vi "DAQSensor-16.vi"() -> ()   [LabVIEW 2016]
uses:
  <vilib>/Utility/error.llb/DialogType.ctl
  PLC-Lab/lib/gusb.dll
panel:
  in  "量程B 5":dbl=100.0
  in  "量程A 5":dbl
  in  "备注 5":string="CH5" caption="CH5"
  in  "选中 5":bool
  in  "量程B 6":dbl=100.0
  in  "量程A 6":dbl
  in  "备注 6":string="CH6" caption="CH6"
  in  "选中 6":bool
  in  "量程B 7":dbl=100.0
  in  "量程A 7":dbl
  in  "备注 7":string="CH7" caption="CH7"
  in  "选中 7":bool
  in  "量程B 8":dbl=100.0
  in  "量程A 8":dbl
  in  "备注 8":string="CH8" caption="CH8"
  in  "选中 8":bool
  in  "量程B 9":dbl=100.0
  in  "量程A 9":dbl
  in  "备注 9":string="CH9" caption="CH9"
  in  "选中 9":bool
  in  "量程B 10":dbl=100.0
  in  "量程A 10":dbl
  in  "备注 10":string="CH10" caption="CH10"
  in  "选中 10":bool
  in  "量程B 11":dbl=100.0
  in  "量程A 11":dbl
  in  "备注 11":string="CH11" caption="CH11"
  in  "选中 11":bool
  in  "量程B 12":dbl=100.0
  in  "量程A 12":dbl
  in  "备注 12":string="CH12" caption="CH12"
  in  "选中 12":bool
  in  "量程B 13":dbl=100.0
  in  "量程A 13":dbl
  in  "备注 13":string="CH13" caption="CH13"
  in  "选中 13":bool
  in  "量程B 14":dbl=100.0
  in  "量程A 14":dbl
  in  "备注 14":string="CH14" caption="CH14"
  in  "选中 14":bool
  in  "量程B 15":dbl=100.0
  in  "量程A 15":dbl
  in  "备注 15":string="CH15" caption="CH15"
  in  "选中 15":bool
  in  "量程B 16":dbl=100.0
  in  "量程A 16":dbl
  in  "备注 16":string="CH16" caption="CH16"
  in  "选中 16":bool
  in  "布尔":bool
  out "采集准备完成":bool
  out "PLC就绪":bool
  out "警告":bool
  out "故障":bool
  out "原位":bool
  out "R0":bool
  out "PLC状态":dbl
  out "实际备注数组":string[](array[string])
  out "通道数":u32
  in  "单位 2":string
  in  "单位 1":string
  in  "单位 3":string
  in  "单位 4":string
  in  "单位 5":string
  in  "单位 6":string
  in  "单位 7":string
  in  "单位 8":string
  in  "单位 9":string
  in  "单位 10":string
  in  "单位 11":string
  in  "单位 12":string
  in  "单位 13":string
  in  "单位 14":string
  in  "单位 15":string
  in  "单位 16":string
  out "系数":sgl[][](array[numeric])
  out "量程B数组":dbl[](array[numeric])
  out "量程A数组":dbl[](array[numeric])
  out "备注数组":string[](array[string])
  out "给采集卡的通道选择":i16
  in  "选项卡控件":enum32{"设置", "数据采集", "历史数据"}(tab)
  in  "最大采集时间(秒)":dbl=5.0 min=0.1 max=15.0
  in  "测试模式选择":enum32{"测试模式1", "测试模式2"}(radio)
  in  "数据存储":bool=TRUE
  in  "量程":u16=10 caption="传感器输出范围"
  in  "通道模式":enum32{"单选选项1", "单选选项2"}(radio)=enum."单选选项2"
  in  "电压电流选择":enum32{"单选选项1", "单选选项2"}(radio)
  in  "产品系列":u16(ring)=1 items=["USB-4000", "USB-2000/1000"]
  in  "传感器单位":string
  in  "数据存储路径":path=path "D:/采集存储/辅助锁力数据"
  in  "传感器输出范围B":dbl=5.0 caption="传感器输出范围"
  in  "传感器输出范围A":dbl caption="传感器输出范围"
  in  "采样率(Sps/s)":u32=500 step=5
  in  "设置生效":bool
  in  "全选":bool
  in  "量程B 2":dbl=100.0
  in  "量程A 2":dbl
  in  "备注 2":string="CH2" caption="CH2"
  in  "选中 2":bool=TRUE
  in  "量程B 1":dbl=100.0
  in  "量程A 1":dbl
  in  "备注 1":string="CH1" caption="CH1"
  in  "选中 1":bool=TRUE
  in  "量程B 3":dbl=100.0
  in  "量程A 3":dbl
  in  "备注 3":string="CH3" caption="CH3"
  in  "选中 3":bool=TRUE
  in  "量程B 4":dbl=100.0
  in  "量程A 4":dbl
  in  "备注 4":string="CH4" caption="CH4"
  in  "选中 4":bool
  in  "转角起点(0.1°)":i32=-350 min=-400 max=400
  in  "转角终点(0.1°)":i32=350 min=200 max=400
  in  "转角速度(转/min)":i32=50 min=10 max=70
  in  "气压设定(0.1MPa)":i32=5 min=2 max=10
  out "测量类型":i32 min=0 max=1
  out "波形图表":sgl[][](graph)
  in  "调用统计信息":bool
  in  "停止":bool
  in  "启动":bool
  in  "转为CSV":bool
  out "波形图表 2":sgl[][](graph)
  in  "历史数据路径":path
  in  "打开":bool
  # "单位"
  # "mA ~              mA"
  # "V ~                 V"
  # "Via Ruiwen"
  # "DAQSensor"
  # "请求原位"
  # "仅启动辅助锁"
  # "通道注释"
  # "传感器量程"
  # "仅USB-2000系列支持差分模式"
  # "~"
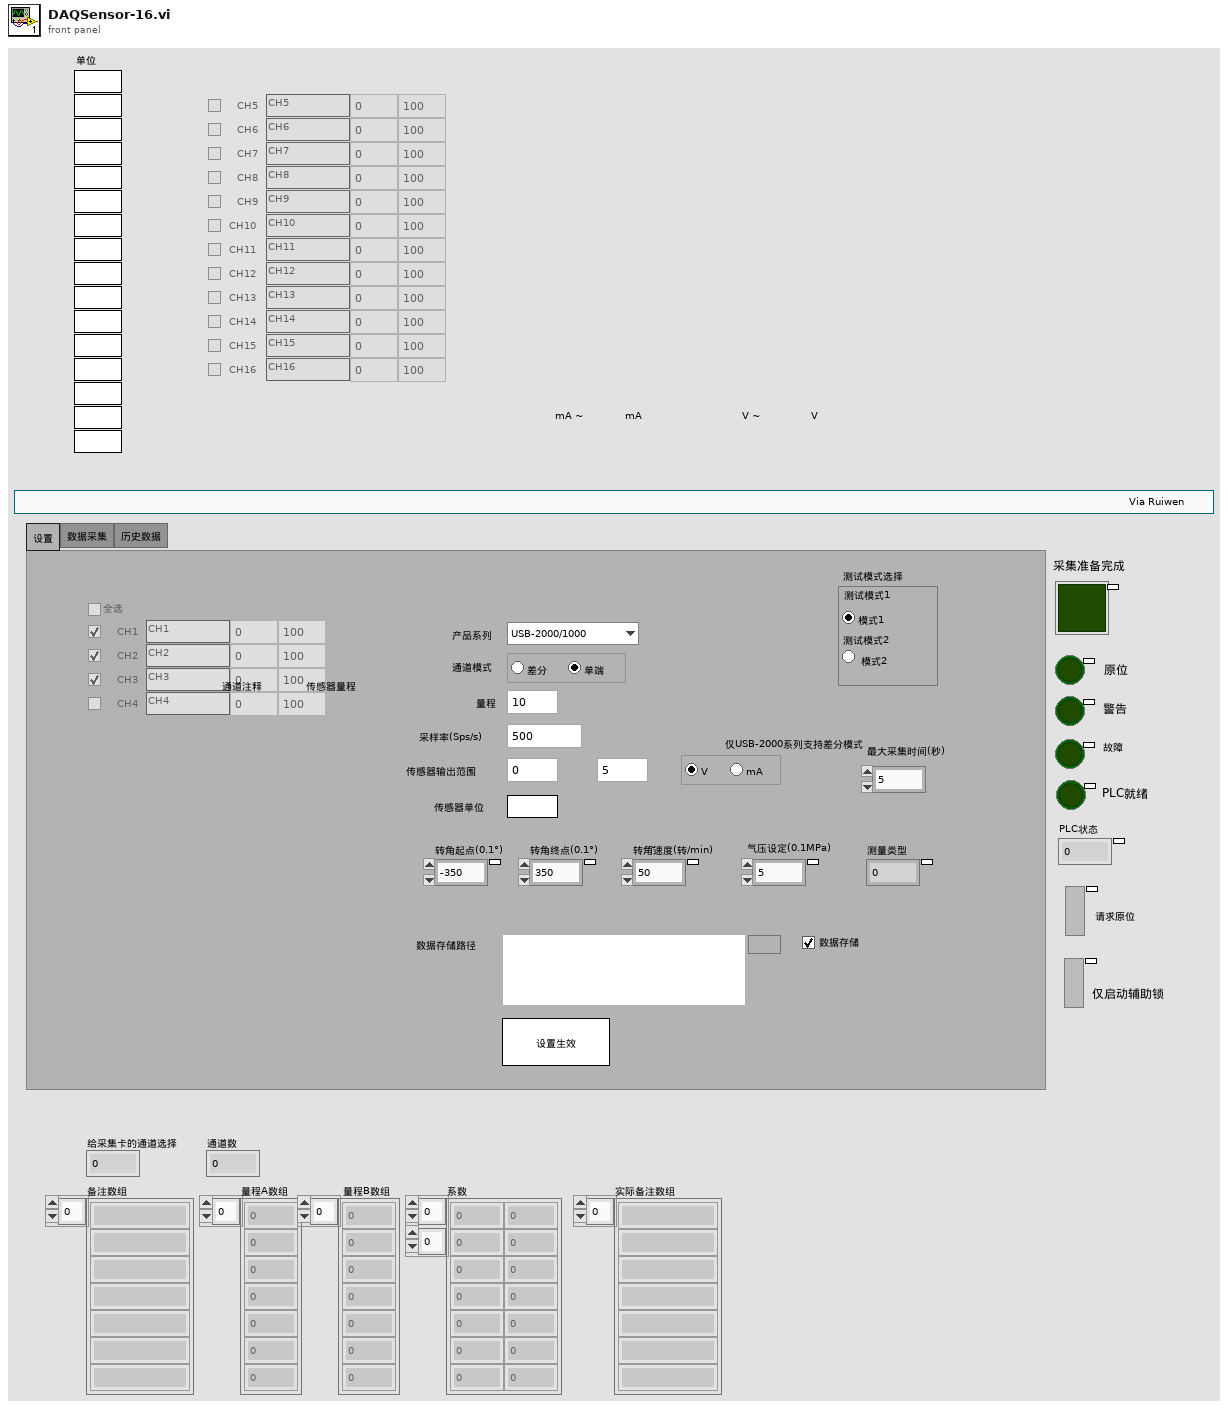
[diagram p1: front panel]
types:
  T1 = enum32{"Bad", "Idle", "Run top level", "Running"}
  T2 = enum8{"Enabled", "Disabled", "Disabled and Grayed Out"}
  T3 = cluster{"seconds since 1Jan1904":timestamp, "采样率":u32, "单位":string, "实际备注数组":string[]}
  T4 = typedef "DialogType.ctl" = u16
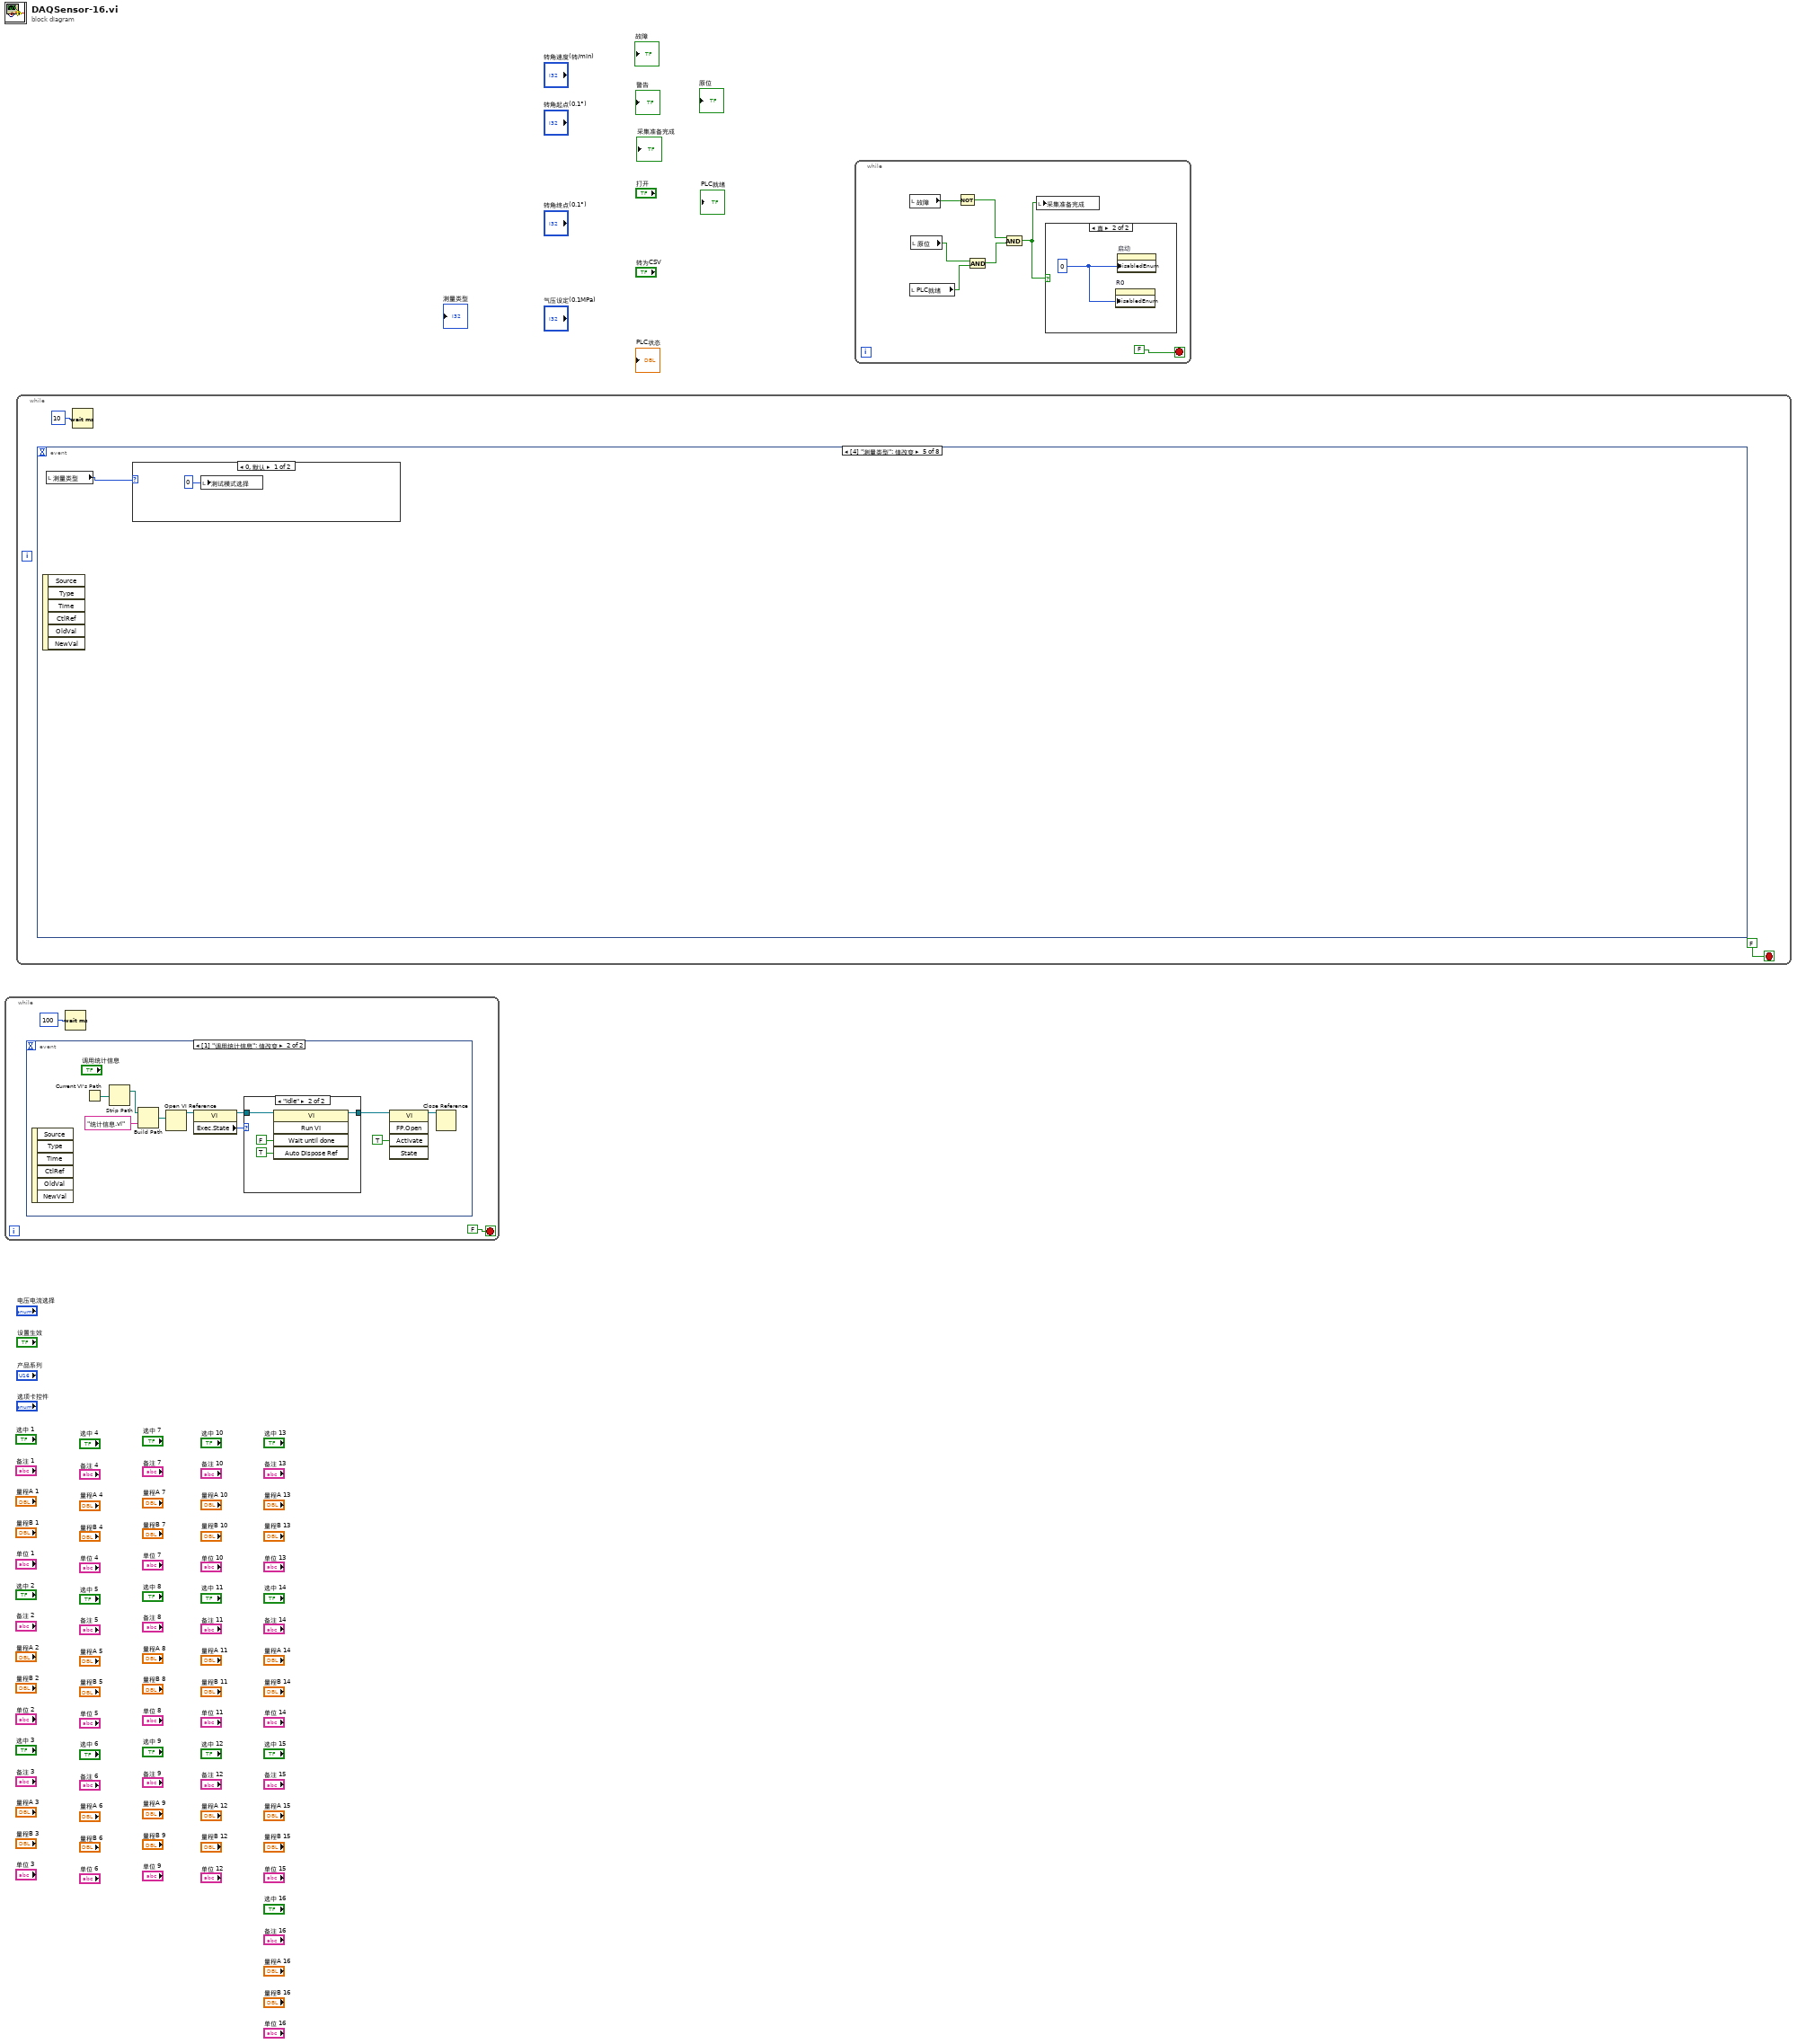
[diagram p0: block diagram]
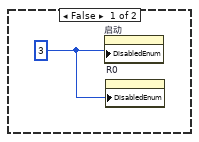
[diagram p2: hidden frame]
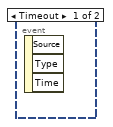
[diagram p3: hidden frame]
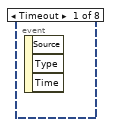
[diagram p5: hidden frame]
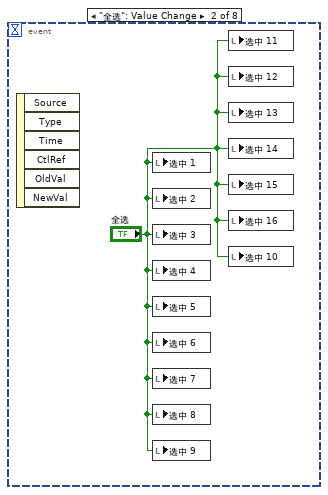
[diagram p6: hidden frame]
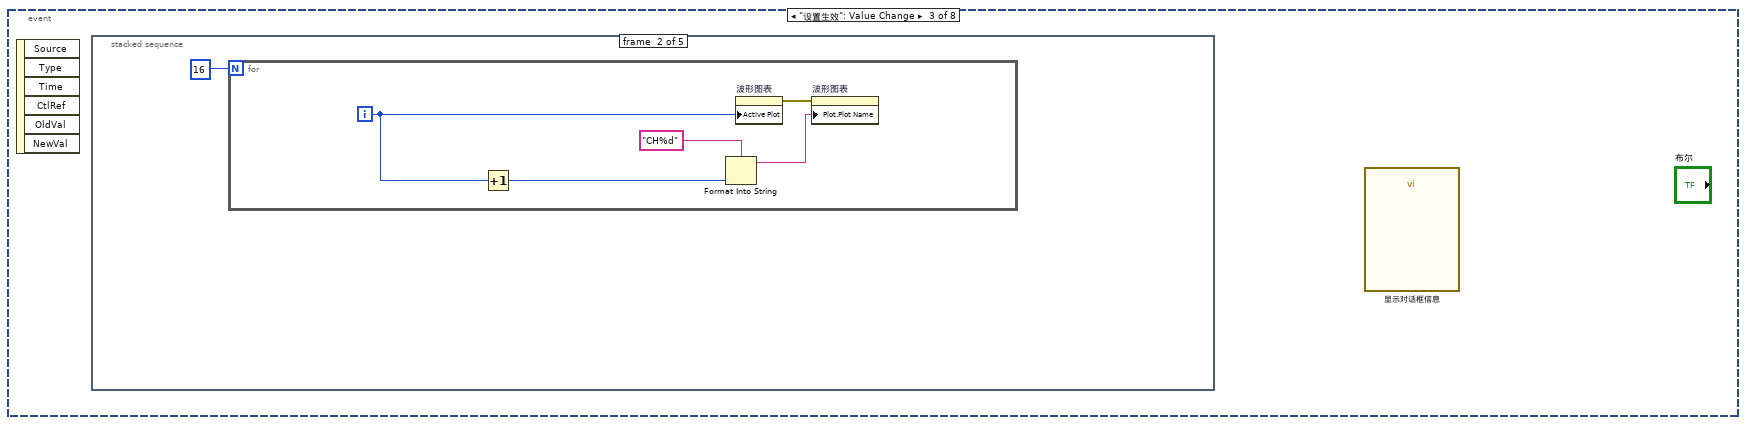
[diagram p7: hidden frame]
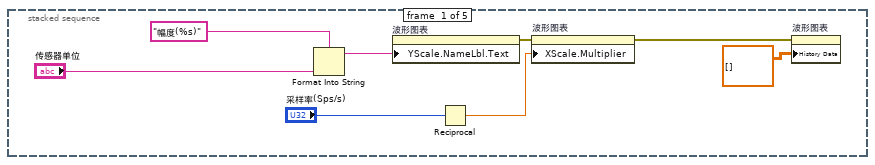
[diagram p8: hidden frame]
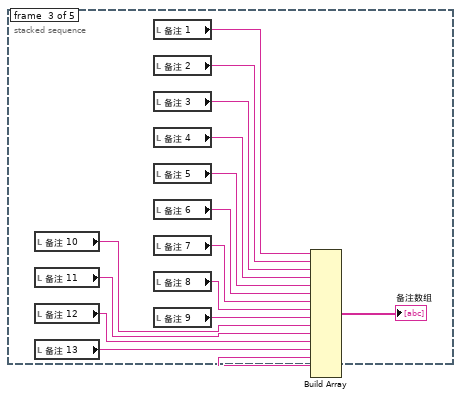
[diagram p9: hidden frame]
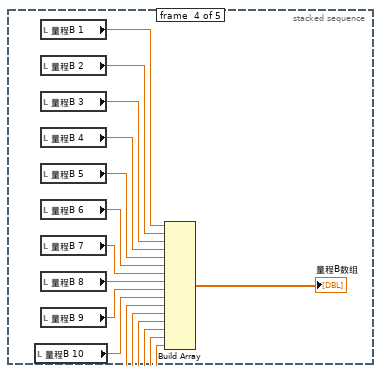
[diagram p10: hidden frame]
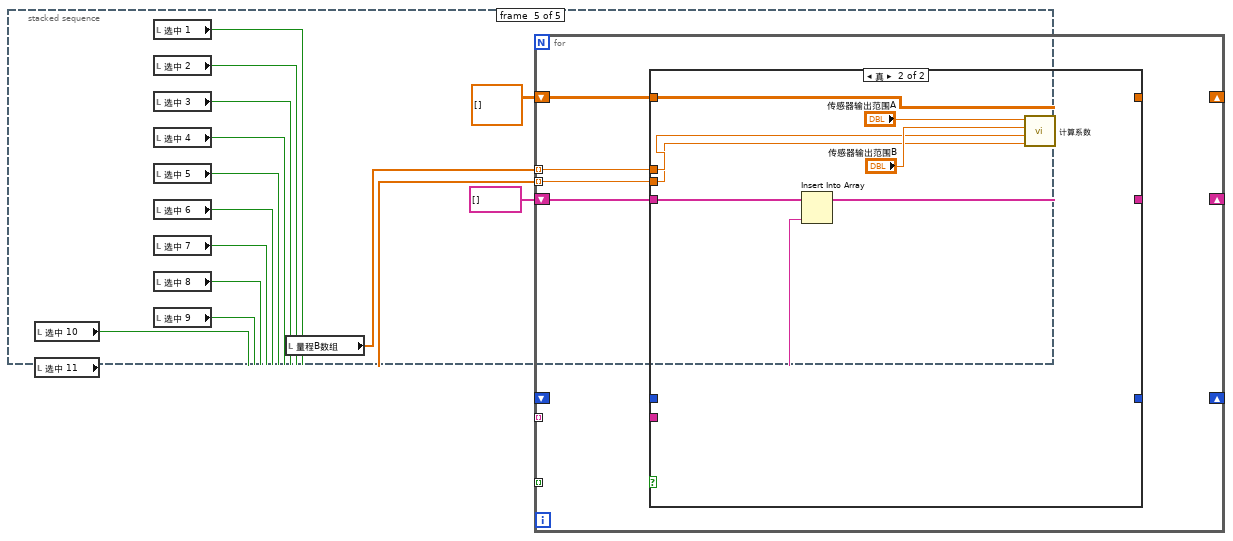
[diagram p11: hidden frame]
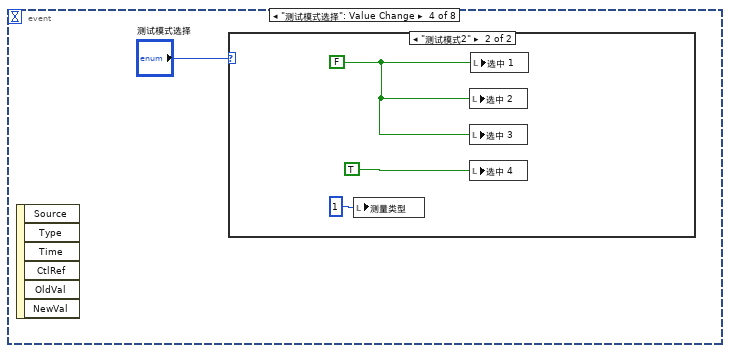
[diagram p13: hidden frame]
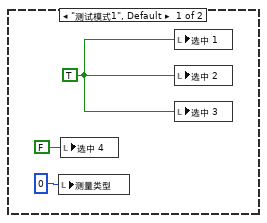
[diagram p14: hidden frame]
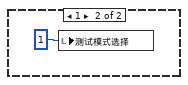
[diagram p15: hidden frame]
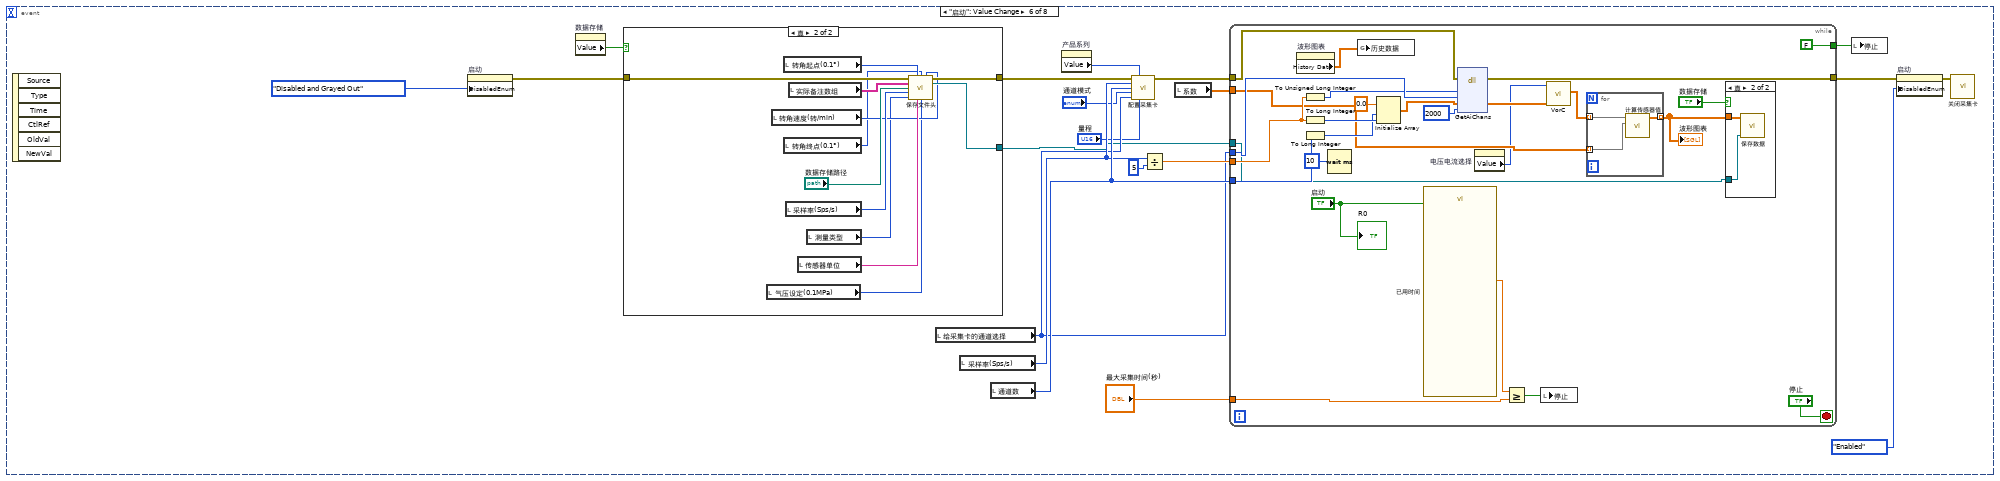
[diagram p16: hidden frame]
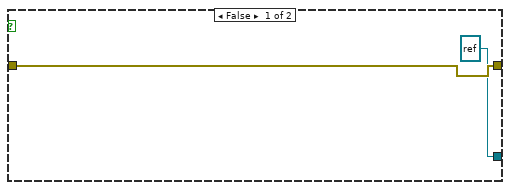
[diagram p17: hidden frame]
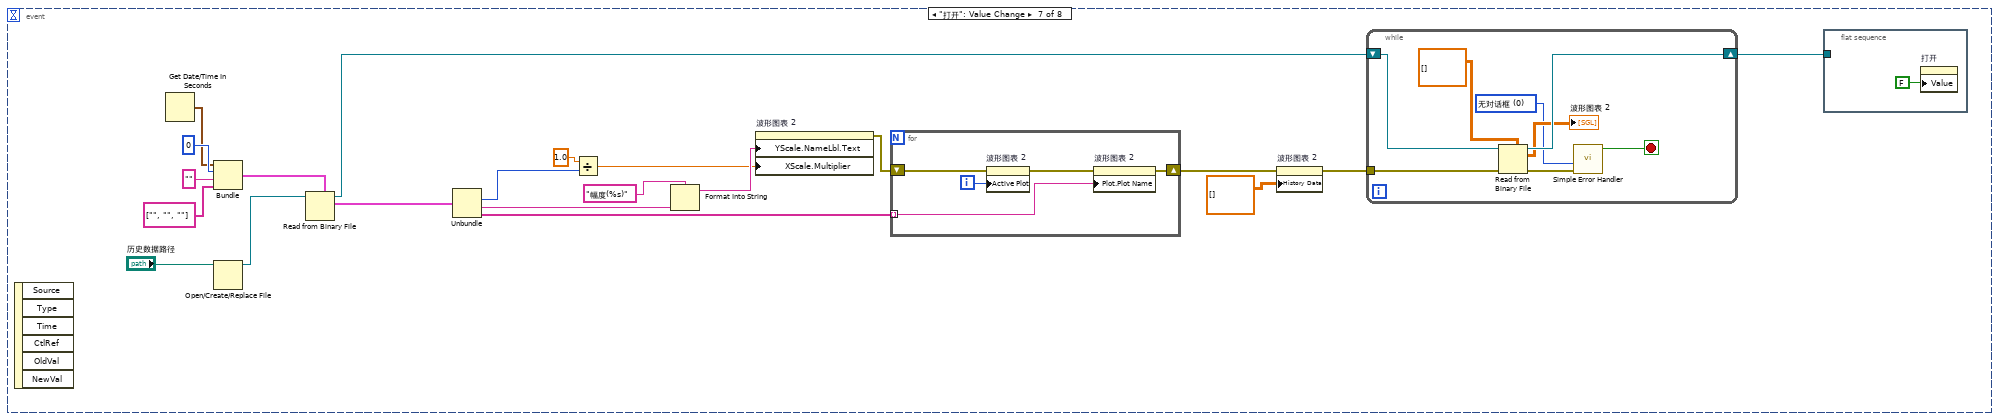
[diagram p19: hidden frame]
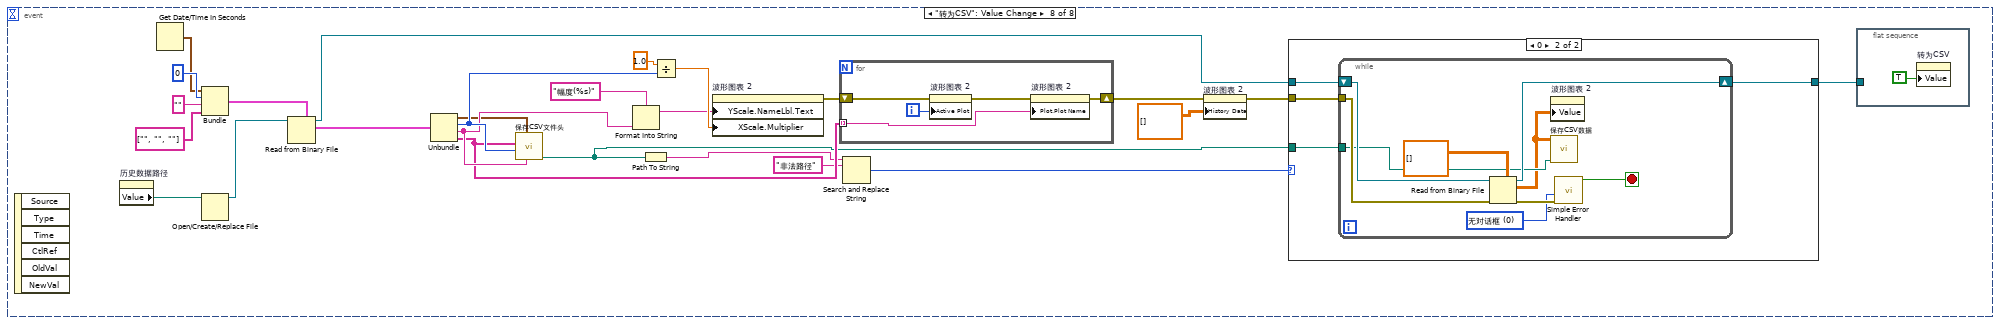
[diagram p20: hidden frame]
diagram:
  n1 = while {
    stop <- FALSE stop-if-true
    n2 = event shown="[1] \"调用统计信息\": 值改变" {
      selector: _ -> [_ _]
      dyn-events: _ -> [_ _]
      timeout: _ -> [_ _]
      event Timeout {
        n3 = event-data() -> ()  [unwired: 1 in, 3 out]
      }
      event "调用统计信息": Value Change {
        n4 = event-data() -> ()  [unwired: 1 in, 6 out]
        n5 = Current VI's Path() -> (path=w3:path)
        n6 = Strip Path(path=w3) -> (stripped path=w4:path)  [unwired: 1 out]
        n7 = Build Path(base path=w4, name or relative path="统计信息.vi" ("名称或相对路径")) -> (appended path=w5:path)
        n8 = Open VI Reference(vi path=w5) -> (vi reference=w6:refnum<vi>)  [unwired: 5 in, 1 out]
        n9 = property class="VI"(reference=w6) -> (reference out=w9:refnum<vi>, "Exec.State"=w7:T1)  [unwired: 1 in, 1 out]
        n10 = case shown="\"Idle\"" w7 {
          tunnel: [w13 w15] -> w8
          tunnel: w9 -> [w13 w14]
          frame "Bad", Default {
          }
          frame "Idle" {
            n11 = invoke class="VI" method="Run VI"(reference=w14, "Wait until done"=FALSE ("结束前等待"), "Auto Dispose Ref"=TRUE ("自动销毁引用")) -> (reference out=w15:refnum<vi>)  [unwired: 2 in, 4 out]
          }
        }
        n12 = invoke class="VI" method="FP.Open"(reference=w8, "Activate"=TRUE ("激活？")) -> (reference out=w11:refnum<vi>)  [unwired: 3 in, 4 out]
        n13 = Close Reference(reference=w11) -> ()  [unwired: 1 in, 1 out]
      }
    }
    n14 = Wait (ms)(milliseconds to wait=u32 100 ("等待时间（毫秒）")) -> ()  [unwired: 1 out]
  }
  n15 = while {
    stop <- FALSE stop-if-true
    n16 = event shown="[4] \"测量类型\": 值改变" {
      selector: _ -> [_ _ _ _ _ _ _ _]
      dyn-events: _ -> [_ _ _ _ _ _ _ _]
      timeout: _ -> [_ _ _ _ _ _ _ _]
      event Timeout {
        n17 = event-data() -> ()  [unwired: 1 in, 3 out]
      }
      event "全选": Value Change {
        n18 = event-data() -> ()  [unwired: 1 in, 6 out]
        n19 = local write "选中 1"("全选") -> ()
        n20 = local write "选中 2"("全选") -> ()
        n21 = local write "选中 3"("全选") -> ()
        n22 = local write "选中 4"("全选") -> ()
        n23 = local write "选中 5"("全选") -> ()
        n24 = local write "选中 6"("全选") -> ()
        n25 = local write "选中 7"("全选") -> ()
        n26 = local write "选中 8"("全选") -> ()
        n27 = local write "选中 9"("全选") -> ()
        n28 = local write "选中 11"("全选") -> ()
        n29 = local write "选中 12"("全选") -> ()
        n30 = local write "选中 13"("全选") -> ()
        n31 = local write "选中 14"("全选") -> ()
        n32 = local write "选中 15"("全选") -> ()
        n33 = local write "选中 16"("全选") -> ()
        n34 = local write "选中 10"("全选") -> ()
      }
      event "设置生效": Value Change {
        n35 = event-data() -> ()  [unwired: 1 in, 6 out]
        n36 = stacked-sequence {
          frame #0 {
            n37 = Format Into String(format string="幅度(%s)" ("格式字符串"), "传感器单位") -> (resulting string=w25:string)  [unwired: 2 in, 1 out]
            n38 = property on="波形图表" class="WFChart (严格)"("YScale.NameLbl.Text"=w25) -> (error out=w21:errorcluster)  [unwired: 2 in, 1 out]
            n39 = Reciprocal(x="采样率(Sps/s)") -> (1/x=w24:dbl)
            n40 = property on="波形图表" class="WFChart (严格)"(error in=w21, "XScale.Multiplier"=w24) -> (error out=w22:errorcluster)  [unwired: 1 in, 1 out]
            n41 = property on="波形图表" class="WFChart (严格)"(error in=w22, "History Data"=dbl[][] [] ("历史数据")) -> ()  [unwired: 1 in, 2 out]
          }
          frame #1 {
            n42 = for {
              N: 16 -> [_]
              i -> [w32]
              n43 = Increment(x=w32) -> (x+1=w33:i32)
              n44 = Format Into String(format string="CH%d" ("格式字符串"), w33) -> (resulting string=w30:string)  [unwired: 2 in, 1 out]
              n45 = property on="波形图表" class="WFChart (严格)"("Active Plot"=w32) -> (error out=w31:errorcluster)  [unwired: 2 in, 1 out]
              n46 = property on="波形图表" class="WFChart (严格)"(error in=w31, "Plot.Plot Name"=w30) -> ()  [unwired: 1 in, 2 out]
            }
          }
          frame #2 {
            n47 = local read "备注 10"() -> (w45:string)
            n48 = local read "备注 11"() -> (w46:string)
            n49 = local read "备注 12"() -> (w47:string)
            n50 = local read "备注 13"() -> (w48:string)
            n51 = local read "备注 14"() -> (w49:string)
            n52 = local read "备注 15"() -> (w50:string)
            n53 = local read "备注 16"() -> (w51:string)
            n54 = local read "备注 1"() -> (w36:string)
            n55 = local read "备注 2"() -> (w37:string)
            n56 = local read "备注 3"() -> (w38:string)
            n57 = local read "备注 4"() -> (w39:string)
            n58 = local read "备注 5"() -> (w40:string)
            n59 = local read "备注 6"() -> (w41:string)
            n60 = local read "备注 7"() -> (w42:string)
            n61 = local read "备注 8"() -> (w43:string)
            n62 = local read "备注 9"() -> (w44:string)
            n63 = Build Array(w36, w37, w38, w39, w40, w41, w42, w43, w44, w45, w46, w47, w48, w49, w50, w51) -> (→"备注数组":string[])
          }
          frame #3 {
            n64 = local read "量程B 10"() -> (w58:dbl)
            n65 = local read "量程B 11"() -> (w57:dbl)
            n66 = local read "量程B 12"() -> (w56:dbl)
            n67 = local read "量程B 13"() -> (w55:dbl)
            n68 = local read "量程B 14"() -> (w54:dbl)
            n69 = local read "量程B 15"() -> (w53:dbl)
            n70 = local read "量程B 16"() -> (w52:dbl)
            n71 = local read "量程A 10"() -> (w79:dbl)
            n72 = local read "量程A 11"() -> (w80:dbl)
            n73 = local read "量程A 12"() -> (w81:dbl)
            n74 = local read "量程A 13"() -> (w82:dbl)
            n75 = local read "量程A 14"() -> (w83:dbl)
            n76 = local read "量程A 15"() -> (w84:dbl)
            n77 = local read "量程A 16"() -> (w85:dbl)
            n78 = local read "量程B 1"() -> (w67:dbl)
            n79 = local read "量程B 2"() -> (w66:dbl)
            n80 = local read "量程B 3"() -> (w65:dbl)
            n81 = local read "量程B 4"() -> (w64:dbl)
            n82 = local read "量程B 5"() -> (w63:dbl)
            n83 = local read "量程B 6"() -> (w62:dbl)
            n84 = local read "量程B 7"() -> (w61:dbl)
            n85 = local read "量程B 8"() -> (w60:dbl)
            n86 = local read "量程B 9"() -> (w59:dbl)
            n87 = local read "量程A 1"() -> (w70:dbl)
            n88 = local read "量程A 2"() -> (w71:dbl)
            n89 = local read "量程A 3"() -> (w72:dbl)
            n90 = local read "量程A 4"() -> (w73:dbl)
            n91 = local read "量程A 5"() -> (w74:dbl)
            n92 = local read "量程A 6"() -> (w75:dbl)
            n93 = local read "量程A 7"() -> (w76:dbl)
            n94 = local read "量程A 8"() -> (w77:dbl)
            n95 = local read "量程A 9"() -> (w78:dbl)
            n96 = Build Array(w67, w66, w65, w64, w63, w62, w61, w60, w59, w58, w57, w56, w55, w54, w53, w52) -> (→"量程B数组":dbl[])
            n97 = Build Array(w70, w71, w72, w73, w74, w75, w76, w77, w78, w79, w80, w81, w82, w83, w84, w85) -> (→"量程A数组":dbl[])
          }
          frame #4 {
            n98 = local read "选中 10"() -> (w104:bool)
            n99 = local read "选中 11"() -> (w103:bool)
            n100 = local read "选中 12"() -> (w102:bool)
            n101 = local read "选中 13"() -> (w101:bool)
            n102 = local read "选中 14"() -> (w100:bool)
            n103 = local read "选中 15"() -> (w99:bool)
            n104 = local read "选中 16"() -> (w98:bool)
            n105 = local read "选中 1"() -> (w113:bool)
            n106 = local read "选中 2"() -> (w112:bool)
            n107 = local read "选中 3"() -> (w111:bool)
            n108 = local read "选中 4"() -> (w110:bool)
            n109 = local read "选中 5"() -> (w109:bool)
            n110 = local read "选中 6"() -> (w108:bool)
            n111 = local read "选中 7"() -> (w107:bool)
            n112 = local read "选中 8"() -> (w106:bool)
            n113 = local read "选中 9"() -> (w105:bool)
            n114 = local read "量程B数组"() -> (w91:dbl[])
            n115 = local read "量程A数组"() -> (w92:dbl[])
            n116 = local read "备注数组"() -> (w93:string[])
            n117 = Build Array(w113, w112, w111, w110, w109, w108, w107, w106, w105, w104, w103, w102, w101, w100, w99, w98) -> (w96:bool[])
            n118 = Boolean Array To Number(Boolean array=w96) -> (number=w97:u32)
            n119 = for {
              tunnel: w96 -> [w123] mode=indexing
              shift-right: [w121] -> w88
              shift-left: u32 0 -> [w122]
              tunnel: w93 -> [w120] mode=indexing
              tunnel: w92 -> [w119] mode=indexing
              tunnel: w91 -> [w118] mode=indexing
              shift-right: [w116] -> w89
              shift-left: dbl[][] [] -> [w117]
              shift-right: [w114] -> w86
              shift-left: string[] [] -> [w115]
              n120 = case shown="真" w123 {
                tunnel: w122 -> [w126 w133]
                tunnel: [w126 w139] -> w121
                tunnel: w120 -> [_ w132]
                tunnel: w119 -> [_ w127]
                tunnel: w118 -> [_ w128]
                tunnel: w117 -> [w125 w137]
                tunnel: [w125 w136] -> w116
                tunnel: w115 -> [w124 w135]
                tunnel: [w124 w134] -> w114
                frame False {
                }
                frame True {
                  n121 = property on="波形图表" class="WFChart (严格)"("Active Plot"=w133) -> (error out=w131:errorcluster)  [unwired: 2 in, 1 out]
                  n122 = Insert Into Array(array=w135, new element=w132) -> (w134:string[])  [unwired: 1 in]
                  n123 = property on="波形图表" class="WFChart (严格)"(error in=w131, "Plot.Plot Name"=w132) -> ()  [unwired: 1 in, 2 out]
                  n124 = call "计算系数.vi"("量程A"=w127, "量程B"=w128, "传感器输出范围B"="传感器输出范围B", "传感器输出范围A"="传感器输出范围A") -> ("系数"=w138:dbl[])  [unwired: 5 in, 2 out]
                  n125 = Increment(x=w133) -> (x+1=w139:u32)
                  n126 = Insert Into Array(array=w137, new element=w138) -> (w136:dbl[][])  [unwired: 2 in]
                }
              }
            }
            "系数" <- w89
            "通道数" <- w88
            "实际备注数组" <- w86
            n127 = To Word Integer(number=w97) -> (16bit integer=→"给采集卡的通道选择":i16)
            n128 = global write "统计全局变量.vi" "实际备注数组"(w86) -> ()
          }
        }
        n129 = call "显示对话框信息"() -> ()  [unwired: 10 in, 2 out]
      }
      event "测试模式选择": Value Change {
        n130 = event-data() -> ()  [unwired: 1 in, 6 out]
        n131 = case shown="\"测试模式2\"" "测试模式选择" {
          frame "测试模式1", Default {
            w143 = TRUE
            n132 = local write "测量类型"(0) -> ()
            n133 = local write "选中 4"(FALSE) -> ()
            n134 = local write "选中 1"(w143) -> ()
            n135 = local write "选中 2"(w143) -> ()
            n136 = local write "选中 3"(w143) -> ()
          }
          frame "测试模式2" {
            w144 = FALSE
            n137 = local write "测量类型"(1) -> ()
            n138 = local write "选中 2"(w144) -> ()
            n139 = local write "选中 3"(w144) -> ()
            n140 = local write "选中 4"(TRUE) -> ()
            n141 = local write "选中 1"(w144) -> ()
          }
        }
      }
      event "测量类型": Value Change {
        n142 = event-data() -> ()  [unwired: 1 in, 6 out]
        n143 = local read "测量类型"() -> (w147:i32)
        n144 = case shown="0, 默认" w147 {
          frame 0, Default {
            n145 = local write "测试模式选择"(0) -> ()
          }
          frame 1 {
            n146 = local write "测试模式选择"(1) -> ()
          }
        }
      }
      event "启动": Value Change {
        n147 = event-data() -> ()  [unwired: 1 in, 6 out]
        n148 = property on="启动" class="Bool"("DisabledEnum"=T2."Disabled and Grayed Out" ("禁用")) -> (error out=w151:errorcluster)  [unwired: 2 in, 1 out]
        n149 = property on="数据存储" class="Bool (严格)"() -> ("Value"=w152:bool)  [unwired: 2 in, 2 out]
        n150 = case shown="真" w152 {
          tunnel: [w171 w183] -> w163
          tunnel: w151 -> [w171 w179]
          tunnel: [refnum<file> refnum ("引用句柄输出") w177] -> w155
          frame False {
          }
          frame True {
            n151 = local read "气压设定(0.1MPa)"() -> (w172:i32)
            n152 = local read "转角速度(转/min)"() -> (w175:i32)
            n153 = local read "转角起点(0.1°)"() -> (w176:i32)
            n154 = local read "转角终点(0.1°)"() -> (w174:i32)
            n155 = local read "采样率(Sps/s)"() -> (w180:u32)
            n156 = local read "实际备注数组"() -> (w182:string[])
            n157 = local read "传感器单位"() -> (w178:string)
            n158 = local read "测量类型"() -> (w173:i32)
            n159 = call "保存文件头.vi"("error in (no error)"=w179, "转角起点"=w176, "转角终点"=w174, "转角速度"=w175, "实际备注数组"=w182, "数据存储路径"="数据存储路径", "采样率"=w180, "测试类型"=w173, "单位"=w178, "气压"=w172) -> ("error out"=w183:errorcluster, "引用句柄输出"=w177:refnum<file>)  [unwired: 3 in, 1 out]
          }
        }
        n160 = local read "给采集卡的通道选择"() -> (w164:i16)
        n161 = local read "采样率(Sps/s)"() -> (w167:u32)
        n162 = local read "通道数"() -> (w168:u32)
        n163 = property on="产品系列" class="Ring (严格)"() -> ("Value"=w156:u16)  [unwired: 2 in, 2 out]
        n164 = call "配置采集卡.vi"("error in"=w163, "产品系列"=w156, "SampleRate"=w167, "通道数"=w168, "ChanMode"="通道模式", "通道选择"=w164, "Range"="量程") -> ("error out"=w169:errorcluster)  [unwired: 8 in]
        n165 = Divide(x=w167, y=u32 5) -> (x/y=w165:dbl)
        n166 = local read "系数"() -> (w161:sgl[][])
        n167 = while {
          tunnel: w169 -> [w204]
          tunnel: w168 -> [w203]
          tunnel: w165 -> [w200]
          tunnel: w164 -> [w201]
          tunnel: [w196] -> w159
          tunnel: w161 -> [w197]
          tunnel: [FALSE] -> w160
          tunnel: w155 -> [w189]
          tunnel: "最大采集时间(秒)" -> [w185]
          stop <- "停止" stop-if-true
          n168 = property on="波形图表" class="WFChart (严格)"() -> ("History Data"=w194:sgl[][])  [unwired: 2 in, 2 out]
          n169 = To Unsigned Long Integer(number=w200) -> (unsigned 32bit integer=w199:u32)
          n170 = To Long Integer(number=w200) -> (32bit integer=w207:i32)
          n171 = To Long Integer(number=w203) -> (32bit integer=w206:i32)
          n172 = Wait (ms)(milliseconds to wait=u32 10 ("等待时间（毫秒）")) -> ()  [unwired: 1 out]
          n173 = global write "统计全局变量.vi" "历史数据"(w194) -> ()
          n174 = Initialize Array(sgl 0.0 ("元素"), w206, w207) -> (w205:sgl[][])
          n175 = call "已用时间"("Reset"="启动") -> ("Elapsed Time (s)"=w187:dbl)  [unwired: 11 in, 7 out]
          n176 = dll-call lib="E:/Camproject/2018/2018.1Labview/PLC-Lab/lib/gusb.dll" fn="GetAiChans"(error in=w204, "Num"=w199, "ChanSel"=w201, "Buf"=w205, "TimeOut"=2000) -> (error out=w196:errorcluster, "Buf"=w193:sgl[][])  [unwired: 6 in, 1 out]
          n177 = property on="电压电流选择" class="RadioBtnsControl (严格)"() -> ("Value"=w191:enum32{"单选选项1", "单选选项2"})  [unwired: 2 in, 2 out]
          n178 = Greater Or Equal?(x=w187, y=w185) -> (x >= y?=w186:bool)
          n179 = local write "停止"(w186) -> ()
          n180 = call "VorC.vi"("Buf"=w193, "电压电流选择"=w191) -> ("Buf 2"=w192:sgl[][])  [unwired: 9 in]
          n181 = for {
            tunnel: w192 -> [w214] mode=indexing
            tunnel: w197 -> [w213] mode=indexing
            tunnel: [w212] -> w190 mode=indexing
            n182 = call "计算传感器值.vi"("系数"=w213, "电压值"=w214) -> ("传感器值"=w212:sgl[])  [unwired: 9 in]
          }
          "波形图表" <- w190
          n183 = case shown="真" "数据存储" {
            tunnel: w190 -> [_ w211]
            tunnel: w189 -> [_ w210]
            frame False {
            }
            frame True {
              n184 = call "保存数据.vi"("数据"=w211, "引用句柄输出"=w210) -> ()  [unwired: 9 in]
            }
          }
          "R0" <- "启动"
        }
        n185 = local write "停止"(w160) -> ()
        n186 = property on="启动" class="Bool"(error in=w159, "DisabledEnum"=T2."Enabled" ("禁用")) -> (error out=w157:errorcluster)  [unwired: 1 in, 1 out]
        n187 = call "关闭采集卡.vi"("error in"=w157) -> ()  [unwired: 10 in, 1 out]
      }
      event "打开": Value Change {
        n188 = event-data() -> ()  [unwired: 1 in, 6 out]
        n189 = Get Date/Time In Seconds() -> (seconds since 1Jan1904=w230:timestamp)
        n190 = Bundle("seconds since 1Jan1904"=w230, "采样率"=u32 0, "单位"="", "实际备注数组"=string[] ["", "", ""]) -> (w229:T3)  [unwired: 1 in]
        n191 = Open/Create/Replace File(file path (use dialog)="历史数据路径") -> (refnum out=w235:refnum<file>)  [unwired: 5 in, 2 out]
        n192 = Read from Binary File(5:w229, 11:w235) -> (2:w226:T3, 3:w234:refnum<file>)  [unwired: 4 in, 2 out]
        n193 = Unbundle(w226) -> ("采样率"=w222:u32, "单位"=w225:string, "实际备注数组"=w220:string[])  [unwired: 1 out]
        n194 = Divide(x=1.0, y=w222) -> (x/y=w221:dbl)
        n195 = Format Into String(format string="幅度(%s)" ("格式字符串"), w225) -> (resulting string=w224:string)  [unwired: 2 in, 1 out]
        n196 = property on="波形图表 2" class="WFChart (严格)"("YScale.NameLbl.Text"=w224, "XScale.Multiplier"=w221) -> (error out=w219:errorcluster)  [unwired: 2 in, 1 out]
        n197 = for {
          tunnel: w220 -> [w248] mode=indexing
          shift-right: [w245] -> w217
          shift-left: w219 -> [w246]
          i -> [w249]
          n198 = property on="波形图表 2" class="WFChart (严格)"(error in=w246, "Active Plot"=w249) -> (error out=w247:errorcluster)  [unwired: 1 in, 1 out]
          n199 = property on="波形图表 2" class="WFChart (严格)"(error in=w247, "Plot.Plot Name"=w248) -> (error out=w245:errorcluster)  [unwired: 1 in, 1 out]
        }
        n200 = property on="波形图表 2" class="WFChart (严格)"(error in=w217, "History Data"=sgl[][] [] ("历史数据")) -> (error out=w216:errorcluster)  [unwired: 1 in, 1 out]
        n201 = while {
          shift-right: [w243] -> w215
          shift-left: w234 -> [w244]
          tunnel: w216 -> [w241]
          stop <- w239 stop-if-true
          w238 = T4 0 items=["无对话框", "确定信息", "继续或停止信息", "确定信息＋警告", "继续/停止+警告"] ("type of dialog (OK msg:1)")
          n202 = Read from Binary File(5:sgl[][] [], 8:w241, 11:w244) -> (0:w240:errorcluster, 2:→"波形图表 2":sgl[][], 3:w243:refnum<file>)  [unwired: 3 in, 1 out]
          n203 = call <vilib>:"Simple Error Handler.vi"("type of dialog (OK msg:1)"=w238, "error in (no error)"=w240) -> ("error?"=w239:bool)  [unwired: 3 in, 4 out]
        }
        n204 = flat-sequence {
          tunnel: w215 -> [_]
          frame #0 {
            n205 = property on="打开" class="Bool (严格)"("Value"=FALSE) -> ()  [unwired: 2 in, 2 out]
          }
        }
      }
      event "转为CSV": Value Change {
        n206 = event-data() -> ()  [unwired: 1 in, 6 out]
        n207 = property on="历史数据路径" class="Path"() -> ("Value"=w255:path)  [unwired: 2 in, 2 out]
        n208 = Get Date/Time In Seconds() -> (seconds since 1Jan1904=w270:timestamp)
        n209 = Bundle("seconds since 1Jan1904"=w270, "采样率"=u32 0, "单位"="", "实际备注数组"=string[] ["", "", ""]) -> (w269:T3)  [unwired: 1 in]
        n210 = Open/Create/Replace File(file path (use dialog)=w255) -> (refnum out=w275:refnum<file>)  [unwired: 5 in, 2 out]
        n211 = Read from Binary File(5:w269, 11:w275) -> (2:w267:T3, 3:w274:refnum<file>)  [unwired: 4 in, 2 out]
        n212 = Unbundle(w267) -> ("seconds since 1Jan1904"=w256:timestamp, "采样率"=w265:u32, "单位"=w264:string, "实际备注数组"=w258:string[])
        n213 = call "保存CSV文件头.vi"("单位"=w264, "当前时间"=w256, "采样率"=w265, "实际备注数组"=w258) -> ("实际存储路径"=w254:path)  [unwired: 6 in, 1 out]
        n214 = Format Into String(format string="幅度(%s)" ("格式字符串"), w264) -> (resulting string=w259:string)  [unwired: 2 in, 1 out]
        n215 = Path To String(path=w254) -> (string=w253:string)
        n216 = Divide(x=1.0, y=w265) -> (x/y=w260:dbl)
        n217 = property on="波形图表 2" class="WFChart (严格)"("YScale.NameLbl.Text"=w259, "XScale.Multiplier"=w260) -> (error out=w263:errorcluster)  [unwired: 2 in, 1 out]
        n218 = for {
          tunnel: w258 -> [w294] mode=indexing
          shift-right: [w291] -> w261
          shift-left: w263 -> [w292]
          i -> [w295]
          n219 = property on="波形图表 2" class="WFChart (严格)"(error in=w292, "Active Plot"=w295) -> (error out=w293:errorcluster)  [unwired: 1 in, 1 out]
          n220 = property on="波形图表 2" class="WFChart (严格)"(error in=w293, "Plot.Plot Name"=w294) -> (error out=w291:errorcluster)  [unwired: 1 in, 1 out]
        }
        n221 = Search and Replace String(input string=w253, search string="非法路径" ("搜索字符串")) -> (number of replacements=w251:i32)  [unwired: 6 in, 3 out]
        n222 = property on="波形图表 2" class="WFChart (严格)"(error in=w261, "History Data"=sgl[][] [] ("历史数据")) -> (error out=w257:errorcluster)  [unwired: 1 in, 1 out]
        n223 = case shown="0" w251 {
          tunnel: w274 -> [_ w281]
          tunnel: w257 -> [_ w280]
          tunnel: w254 -> [_ w279]
          tunnel: [refnum<file> refnum ("refnum out") w278] -> w250
          frame 1, Default {
          }
          frame 0 {
            n224 = while {
              shift-right: [w289] -> w278
              shift-left: w281 -> [w290]
              tunnel: w280 -> [w288]
              tunnel: w279 -> [w283]
              stop <- w286 stop-if-true
              w285 = T4 0 items=["无对话框", "确定信息", "继续或停止信息", "确定信息＋警告", "继续/停止+警告"] ("type of dialog (OK msg:1)")
              n225 = Read from Binary File(5:sgl[][] [], 8:w288, 11:w290) -> (0:w287:errorcluster, 2:w282:sgl[][], 3:w289:refnum<file>)  [unwired: 3 in, 1 out]
              n226 = property on="波形图表 2" class="WFChart (严格)"("Value"=w282) -> ()  [unwired: 2 in, 2 out]
              n227 = call "保存CSV数据.vi"("路径"=w283, "数据"=w282) -> ()  [unwired: 10 in]
              n228 = call <vilib>:"Simple Error Handler.vi"("type of dialog (OK msg:1)"=w285, "error in (no error)"=w287) -> ("error?"=w286:bool)  [unwired: 3 in, 4 out]
            }
          }
        }
        n229 = flat-sequence {
          tunnel: w250 -> [_]
          frame #0 {
            n230 = property on="转为CSV" class="Bool (严格)"("Value"=TRUE) -> ()  [unwired: 2 in, 2 out]
          }
        }
      }
    }
    n231 = Wait (ms)(milliseconds to wait=u32 10 ("等待时间（毫秒）")) -> ()  [unwired: 1 out]
  }
  n232 = while {
    stop <- FALSE stop-if-true
    n233 = local read "故障"() -> (w301:bool)
    n234 = local read "PLC就绪"() -> (w300:bool)
    n235 = local read "原位"() -> (w299:bool)
    n236 = Not(x=w301) -> (.not. x?=w298:bool)
    n237 = And(x=w299, y=w300) -> (x .and. y?=w297:bool)
    n238 = And(x=w298, y=w297) -> (x .and. y?=w296:bool)
    n239 = local write "采集准备完成"(w296) -> ()
    n240 = case shown="真" w296 {
      frame False {
        w303 = 3
        n241 = property on="启动" class="Bool"("DisabledEnum"=w303) -> ()  [unwired: 2 in, 2 out]
        n242 = property on="R0" class="Bool (严格)"("DisabledEnum"=w303) -> ()  [unwired: 2 in, 2 out]
      }
      frame True {
        w304 = 0
        n243 = property on="R0" class="Bool (严格)"("DisabledEnum"=w304) -> ()  [unwired: 2 in, 2 out]
        n244 = property on="启动" class="Bool"("DisabledEnum"=w304) -> ()  [unwired: 2 in, 2 out]
      }
    }
  }
